vi "Self Shut Down.vi"(11 "Display Actor in":refnum<class "Display Actor.lvclass">) -> (3 "Display Actor out":refnum<class "Display Actor.lvclass">)   [LabVIEW 2024, in "Display Actor.lvclass"]
uses:
  Display Actor.lvclass
  Ancestor Class/Message/Message.lvclass
  Ancestor Class/Message/Type Def/CMD Type.ctl
  Ancestor Class/Message/Type Def/General CMD.ctl
  Ancestor Class/Actor/System Actor/System Actor.lvclass/System Actor.ctl
  Ancestor Class/Message/Message.lvclass/Message.ctl
  Ancestor Class/Message/Public Data/Write CMD Type.vi
  Ancestor Class/Message/Public Data/Write General CMD.vi
  Ancestor Class/Actor/System Actor/Public Data/Read ID.vi
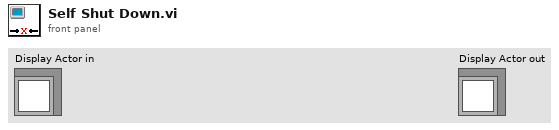
[diagram p1: front panel]
types:
  T1 = typedef "General CMD.ctl" = enum16{"None", "Stop", "Abort", "Running Task", "Running Batch Tasks", "Task Self Running", "Emergency Stop", "Subscribe", "UnSubscribe", "Pause", "Receive Parameters", "Active"}
  T2 = typedef "CMD Type.ctl" = enum16{"None", "General CMD", "1st CMD", "2nd CMD", "3rd CMD", "4th CMD", "5th CMD", "6th CMD", "7th CMD"}
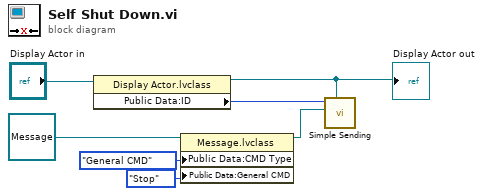
[diagram p0: block diagram]
diagram:
  n1 = property class="Display Actor.lvclass"(reference="Display Actor in") -> (reference out=w6:refnum<class "Display Actor.lvclass">, "Public Data:ID"=w5:i64)  [unwired: 1 in, 1 out]
  "Display Actor out" <- w6
  n2 = property class="Message.lvclass"(reference=refnum<class "Message.lvclass"> refnum ("Message.lvclass"), "Public Data:CMD Type"=CMD_Type."General CMD" ("CMD Type"), "Public Data:General CMD"=General_CMD."Stop" ("General CMD")) -> (reference out=w1:refnum<class "Message.lvclass">)  [unwired: 1 in, 1 out]
  n3 = call "Simple Sending.vi"("System Actor In"=w6, "Message In"=w1, "ID In"=w5) -> ()  [unwired: 9 in]
